vi "Log Data.vi"(8 "error in (no error)":errorcluster, 10 "Data Queue":refnum<queue>, 11 "Logging Configuration":T1) -> (0 "error out":errorcluster)   [LabVIEW 2025, in "Logging.lvlib"]
doc: "This VI uses the TDMS Write function to write data to a TDMS file."
uses:
  Logging.lvlib
  Logging Configuration.ctl
panel:
  # "Simulator Fit"
  # "Empirical Fit"
  # "="
  # "P"
  # "* X"
  # "P"
  # "="
  # "* X"
  # "drop"
  # "drop"
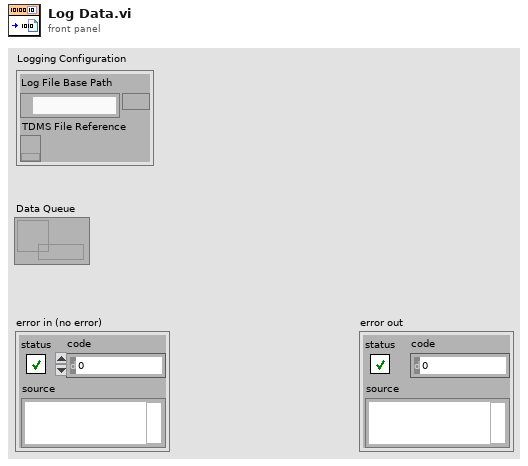
[diagram p1: front panel]
types:
  T1 = typedef "Logging.lvlib/Logging Configuration.ctl" = cluster{"Log File Base Path":path, "TDMS File Reference":refnum<k34>}
  T2 = cluster{"Waveform":waveform(dbl), "Design Results":cluster{"Model Validation: Simulated vs. Empirical Airflow Data":cluster{dbl[], dbl[]}[], "Amplitude - Empirical":string, "Power - Empirical":string, "Amplitude - Sim":string, "Power - Sim":string, "Flow Type":u32, "Optimized Inlet \nOrifice Diameter (in)":dbl, "Flow Type Name":string}}
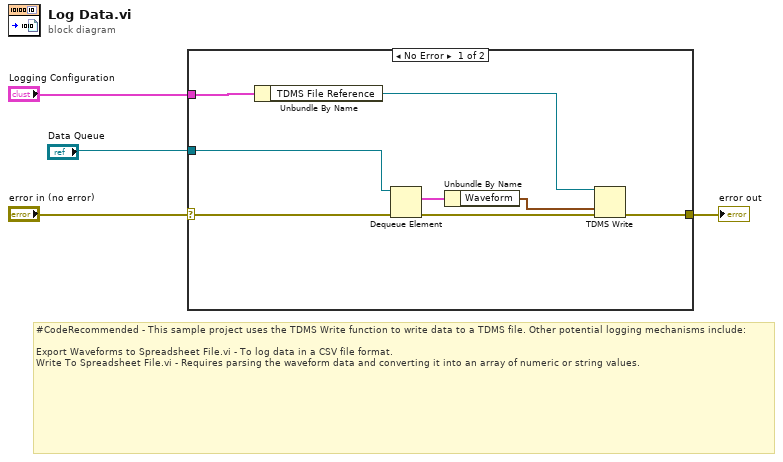
[diagram p0: block diagram]
diagram:
  # "#CodeRecommended - This sample project uses the TDMS Write function to write data to a TDMS file. Other potential logging mechanisms include:\n\nExport Waveforms to Spreadsheet File.vi - To log data in a CSV file format.\nWrite To Spreadsheet File.vi - Requires parsing the waveform data and converting it into an array of numeric or string values."
  n1 = case shown="No Error" "error in (no error)" {
    selector: "error in (no error)" -> [w10 w13]
    tunnel: "Logging Configuration" -> [w12 _]
    tunnel: "Data Queue" -> [w9 _]
    tunnel: [w11 w13] -> w3
    frame No Error {
      n2 = Unbundle By Name(w12) -> ("TDMS File Reference"=w7:refnum<k34>)
      n3 = Dequeue Element(queue=w9, error in (no error)=w10) -> (element=w6:T2, error out=w8:errorcluster)  [unwired: 1 in, 2 out]
      n4 = Unbundle By Name(w6) -> ("Waveform"=w5:waveform(dbl))
      n5 = TDMS Write(0:w7, 9:w5, 11:w8) -> (15:w11:errorcluster)  [unwired: 3 in, 3 out]
    }
    frame Error {
    }
  }
  "error out" <- w3
